vi "Write Variable.vi"(8 "error in (no error)":errorcluster, 9 "Memory Cell":T1, 10 "Variable Name":string, 11 "gScript Interpreter in":refnum<class "gScript Interpreter.lvclass">) -> (0 "error out":errorcluster, 3 "gScript Interpreter out":refnum<class "gScript Interpreter.lvclass">)   [LabVIEW 2023, in "gScript Interpreter.lvclass"]
uses:
  gScript Interpreter.lvclass
  Type Definitions/Memory Cell.ctl
  Type Definitions/Memory Cell Type Enum.ctl
  Type Definitions/Variable.ctl
  gScript Interpreter.lvclass/gScript Interpreter.ctl
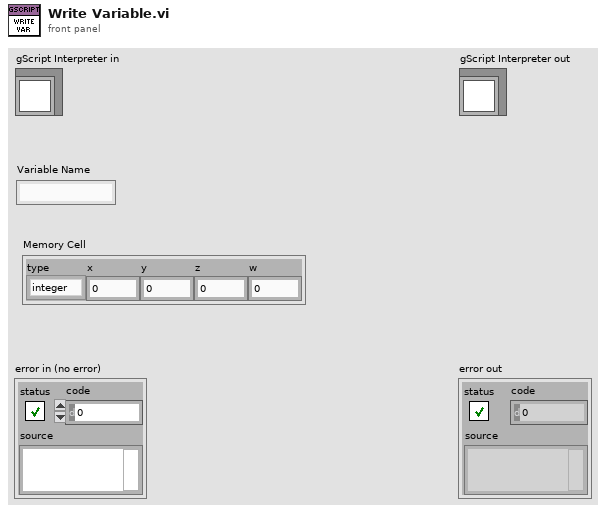
[diagram p1: front panel]
types:
  T1 = typedef "Memory Cell.ctl" = cluster{"type":T2, "x":dbl, "y":dbl, "z":dbl, "w":dbl}
  T2 = typedef "Memory Cell Type Enum.ctl" = enum16{"integer", "float", "vector", "rotation"}
  T3 = typedef "Variable.ctl" = cluster{"Variable Name":string, "Memory Cell":T1}
  T4 = typedef "Stack Frame.ctl" = cluster{"Variable Table":T5, "Return Pointer":i32, "Return Bindings":string[]}
  T5 = typedef "Variable Table.ctl" = T3[]
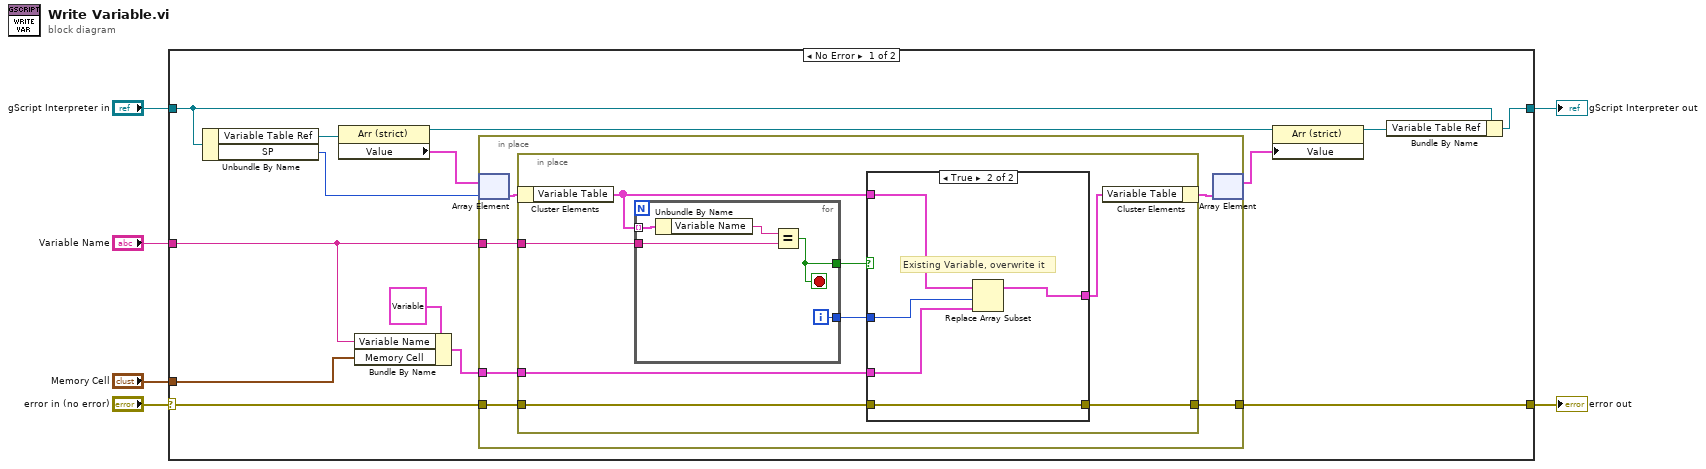
[diagram p0: block diagram]
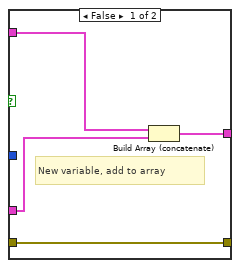
[diagram p2: hidden frame]
diagram:
  n1 = case shown="No Error" "error in (no error)" {
    selector: "error in (no error)" -> [w19 w50]
    tunnel: [w18 w50] -> w5
    tunnel: [w10 w49] -> w3
    tunnel: "gScript Interpreter in" -> [w11 w49]
    tunnel: "Variable Name" -> [w16 _]
    tunnel: "Memory Cell" -> [w15 _]
    frame No Error {
      n2 = Unbundle By Name(w11) -> ("Variable Table Ref"=w20:refnum<vi>, "SP"=w8:i32)
      n3 = property class="Arr (strict)"(reference=w20) -> (reference out=w13:refnum<vi>, "Value"=w9:T4[])  [unwired: 1 in, 1 out]
      n4 = Bundle By Name(cluster=T3 {"Variable Name"="", "Memory Cell"={"type"=enum."integer", "x"=0.0, "y"=0.0, "z"=0.0, "w"=0.0}} ("Cluster"), "Variable Name"=w16, "Memory Cell"=w15) -> (w14:T3)
      n5 = in-place {
        in-place-border: w19 -> [w26]
        in-place-border: [w25] -> w18
        in-place-border: w16 -> [w24]
        in-place-border: w14 -> [w23]
        n6 = in-place-array #1(w9, w8) -> (w22:T4)
        n7 = in-place {
          in-place-border: w26 -> [w33]
          in-place-border: [w32] -> w25
          in-place-border: w24 -> [w30]
          in-place-border: w23 -> [w29]
          n8 = in-place-cluster #2(w22) -> ("Variable Table"=w28:T5)
          n9 = for {
            tunnel: w28 -> [w45] mode=indexing
            tunnel: w30 -> [w47]
            tunnel: [w46] -> w34
            tunnel: [w44] -> w31
            i -> [w44]
            stop <- w46 stop-if-true
            n10 = Unbundle By Name(w45) -> ("Variable Name"=w48:string)
            n11 = Equal?(x=w48, y=w47) -> (x = y?=w46:bool)
          }
          n12 = case shown="True" w34 {
            tunnel: w33 -> [w38 w43]
            tunnel: [w38 w43] -> w32
            tunnel: w28 -> [w37 w42]
            tunnel: w31 -> [_ w40]
            tunnel: [w35 w41] -> w27
            tunnel: w29 -> [w36 w39]
            frame False {
              # "New variable, add to array"
              n13 = Build Array (concatenate)(w37, w36) -> (w35:T5)
            }
            frame True {
              # "Existing Variable, overwrite it"
              n14 = Replace Array Subset(array=w42, new element=w39, index=w40) -> (w41:T5)
            }
          }
          n15 = in-place-cluster #2("Variable Table"=w27) -> (w21:T4)
        }
        n16 = in-place-array #1(w21) -> (w7:T4[])  [unwired: 1 out]
      }
      n17 = property class="Arr (strict)"(reference=w13, "Value"=w7) -> (reference out=w12:refnum<vi>)  [unwired: 1 in, 1 out]
      n18 = Bundle By Name(cluster=w11, "Variable Table Ref"=w12) -> (w10:refnum<class "gScript Interpreter.lvclass">)
    }
    frame Error {
    }
  }
  "error out" <- w5
  "gScript Interpreter out" <- w3
